vi "p2.vi"() -> ()   [LabVIEW 2021, in "d4.lvlib"]
uses:
  d4.lvlib
  e7f17c8a-1ff6-4748-8bb6-0c6253178857.vi
  <vilib>/Analysis/1siggen.llb/Ramp Pattern by Delta.vi
  AOC/AOC.lvlib
  <vilib>/Analysis/NI_AALBase.lvlib
panel:
  in  "Example":string
  in  "Example":bool
  out "Answer":i64
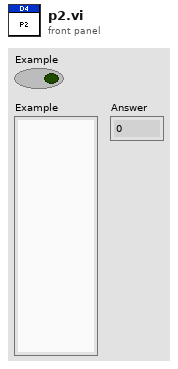
[diagram p1: front panel]
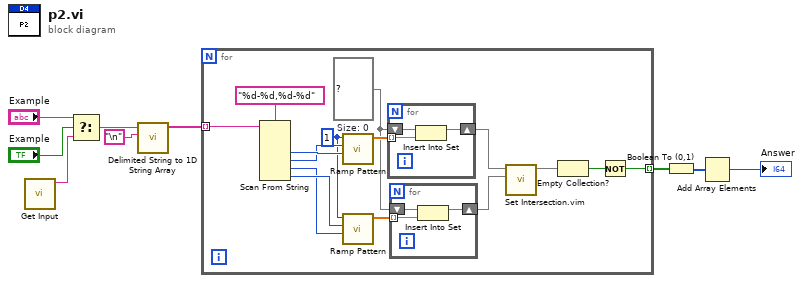
[diagram p0: block diagram]
diagram:
  n1 = call "Get Input.vi"() -> ("Input"=w9:string)  [unwired: 11 in]
  n2 = Select(t="Example", s="Example", f=w9) -> (s? t:f=w8:string)
  n3 = call <vilib>:"Delimited String to 1D String Array.vi"("delimiter"="\n", "delimited string"=w8) -> ("string array"=w2:string[])  [unwired: 9 in]
  n4 = for {
    tunnel: w2 -> [w24] mode=indexing
    tunnel: [w10] -> w4 mode=indexing
    w18 = set{i64} {}  # Size: 0
    w17 = i64 1 ("delta")
    n5 = Scan From String(format string="%d-%d,%d-%d", input string=w24) -> (output 1=w22:i32, output 2=w21:i32, output 3=w15:i32, output 4=w16:i32)  [unwired: 6 in, 3 out]
    n6 = call-poly <vilib>:"Ramp Pattern.vi"("start"=w22, "end"=w21, "delta"=w17) -> ("Ramp Pattern"=w20:dbl[])  [unwired: 6 in, 2 out]
    n7 = call-poly <vilib>:"Ramp Pattern.vi"("start"=w15, "end"=w16, "delta"=w17) -> ("Ramp Pattern"=w19:dbl[])  [unwired: 6 in, 2 out]
    n8 = for {
      tunnel: w20 -> [w30] mode=indexing
      shift-right: [w29] -> w14
      shift-left: w18 -> [w28]
      n9 = Insert Into Set(10:w30, 11:w28) -> (3:w29:set{i64})  [unwired: 1 out]
    }
    n10 = for {
      tunnel: w19 -> [w27] mode=indexing
      shift-right: [w26] -> w13
      shift-left: w18 -> [w25]
      n11 = Insert Into Set(10:w27, 11:w25) -> (3:w26:set{i64})  [unwired: 1 out]
    }
    n12 = call "Set Intersection.vim"("set 2"=w13, "set 1"=w14) -> ("intersection"=w12:set{i64})  [unwired: 9 in]
    n13 = Empty Collection?(1:w12) -> (0:w11:bool)
    n14 = Not(x=w11) -> (.not. x?=w10:bool)
  }
  n15 = Boolean To (0,1)(Boolean=w4) -> (0, 1=w3:i16[])
  n16 = Add Array Elements(numeric array=w3) -> (sum=→"Answer":i16)
